vi "Find Edge.vi"(8 "error in":errorcluster, 9 "input cluster":T1, 11 "Gantry In":refnum<k24>) -> (0 "error out":errorcluster, 3 "Gantry Out":refnum<k24>)   [LabVIEW 2021, in "Component Tray.lvclass"]
uses:
  Workspace/Component/Component Tray.lvclass
  C:/Program Files (x86)/Aerotech/A3200/LabVIEW/2010/Bin/Aerotech.A3200.dll
  Program Files (x86)/Aerotech/A3200/LabVIEW/2010/Bin/Aerotech.A3200.dll
  Workspace/Component/Find Component.ctl
  Camera/Machine Vision.ctl
  A3200.lvclass
  Camera/Camera.lvclass
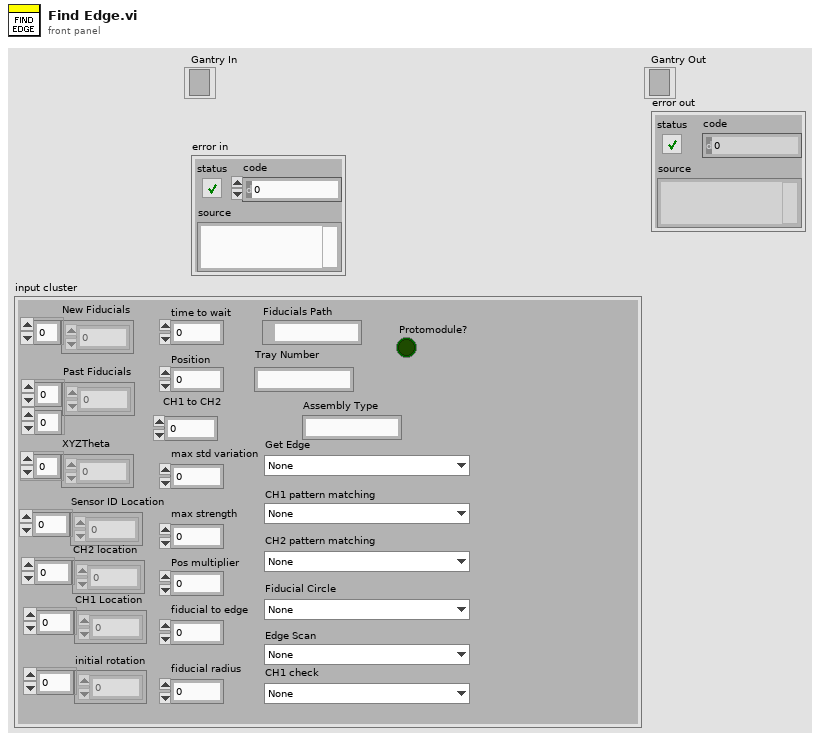
[diagram p1: front panel]
types:
  T1 = typedef "Component Tray.lvclass/Find Component.ctl" = cluster{"New Fiducials":dbl[], "Past Fiducials":dbl[][], "XYZTheta":dbl[], "Fiducials Path":path, "Position":i32, "CH1 Location":dbl[], "Sensor ID Location":dbl[], "initial rotation":dbl[], "CH2 location":dbl[], "max std variation":dbl, "max strength":dbl, "CH2 pattern matching":T2, "Fiducial Circle":T2, "Get Edge":T2, "Pos multiplier":dbl, "time to wait":u32, "fiducial to edge":dbl, "Protomodule?":bool, "Assembly Type":string, "CH1 to CH2":dbl, "Tray Number":string, "fiducial radius":dbl, "4 fiducials?":bool, "CH1 check":T2, "Edge Scan":T2, "CH1 pattern matching":T2, "Sensor Thickness":dbl}
  T2 = typedef "Camera.lvclass/Machine Vision.ctl" = enum16{"None", "Assembly Tray Circle", "Assembly Tray Fiducial", "Partial Hexaboard", "sensor edge init", "HB edge init", "sensor edge pos1", "sensor edge pos2", "HB edge pos1", "HB edge pos2", "Sensor CH1-2", "HB CH1", "HB CH2", "V3 Sensor Circle", "Hexaboard Circle", "sensor CH1 check", "HB CH1 check "}
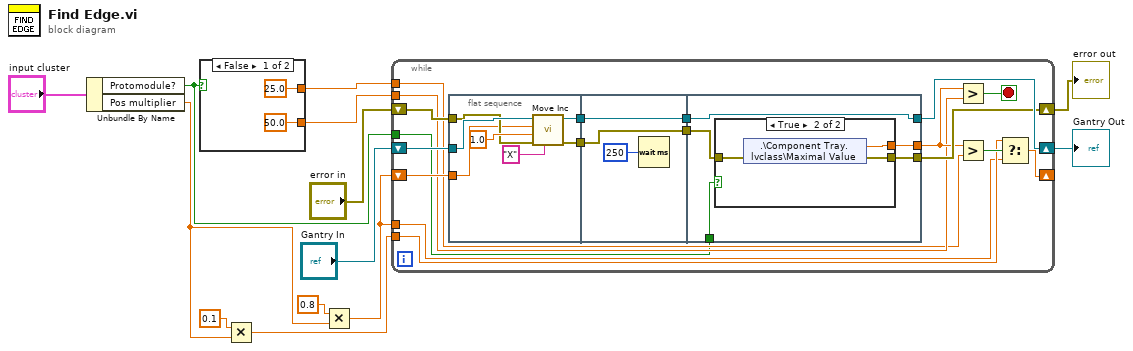
[diagram p0: block diagram]
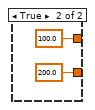
[diagram p2: hidden frame]
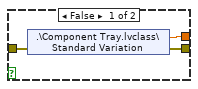
[diagram p3: hidden frame]
diagram:
  n1 = Unbundle By Name("input cluster") -> ("Protomodule?"=w2:bool, "Pos multiplier"=w1:dbl)
  n2 = case shown="False" w2 {
    tunnel: [sgl 50.0 ("y") sgl 200.0 ("y")] -> w4
    tunnel: [sgl 25.0 ("y") sgl 100.0 ("y")] -> w3
    frame False {
    }
    frame True {
    }
  }
  n3 = Multiply(x=0.1, y=w1) -> (x*y=w6:dbl)
  n4 = Multiply(x=0.8 ("Distance"), y=w1) -> (x*y=w7:dbl)
  n5 = while {
    shift-right: [w32] -> w10
    shift-left: "Gantry In" -> [w35]
    shift-right: [w28] -> w8
    shift-left: "error in" -> [w31]
    shift-right: [w23] -> _
    shift-left: w7 -> [w26]
    tunnel: w7 -> [w24]
    tunnel: w6 -> [w25]
    tunnel: w4 -> [w20]
    tunnel: w3 -> [w19]
    tunnel: w2 -> [w18]
    stop <- w22 stop-if-true
    n6 = flat-sequence {
      tunnel: w35 -> [w40]
      tunnel: [w39] -> w33
      tunnel: w31 -> [w38]
      tunnel: [w37] -> w29
      tunnel: w26 -> [w36]
      tunnel: [w45] -> w34
      tunnel: w33 -> [w45]
      tunnel: [w44] -> w30
      tunnel: w29 -> [w44]
      tunnel: [w50] -> w32
      tunnel: w34 -> [w50]
      tunnel: w30 -> [w48]
      tunnel: [w47] -> w28
      tunnel: [w49] -> w21
      tunnel: w18 -> [w46]
      frame #0 {
        n7 = call "Move Inc.vi"("Axis"="X", "error in (no error)"=w38, "Speed"=1.0, "Distance"=w36, "Gantry In"=w40) -> ("error out"=w37:errorcluster, "Gantry Out"=w39:refnum<k24>)  [unwired: 5 in]
      }
      frame #1 {
        n8 = Wait (ms)(milliseconds to wait=u32 250) -> ()  [unwired: 1 out]
      }
      frame #2 {
        n9 = case shown="True" w46 {
          tunnel: [w52 w56] -> w49
          tunnel: w48 -> [w53 w55]
          tunnel: [w51 w54] -> w47
          frame False {
            n10 = shared-variable ".\\Component Tray.lvclass\\Standard Variation"(error in=w53) -> (w52:sgl, error out=w51:errorcluster)
          }
          frame True {
            n11 = shared-variable ".\\Component Tray.lvclass\\Maximal Value"(error in=w55) -> (w56:sgl, error out=w54:errorcluster)
          }
        }
      }
    }
    n12 = Greater?(x=w21, y=w20) -> (0:w22:bool)
    n13 = Greater?(x=w21, y=w19) -> (0:w27:bool)
    n14 = Select(t=w25, s=w27, f=w24) -> (s? t:f=w23:dbl)
  }
  "Gantry Out" <- w10
  "error out" <- w8
